vi "反应性计算.vi"(0 "首循环？":bool, 1 "λi*Ci(0)":sgl[][](array[numeric])=[[82.89727, 82.892685, 82.89905, 82.885956]], 3 "N(0)IN":sgl[](array[numeric]), 5 "βi":sgl[](array[numeric])=[0.000176, 0.001258, 0.001139, 0.002309, 0.000791, 0.000288], 7 "λi":sgl[](array[numeric])=[0.0125, 0.0306, 0.1167, 0.3133, 1.217, 3.266], 9 "中子寿命":sgl=2.3e-05, 11 "源强":sgl[](array[numeric]), 12 "采集间隔":sgl=0.05, 13 "中子注量率":dbl[](array[numeric])=[82.89727020263672, 82.89268493652344, 82.8990478515625, 82.88595581054688]) -> (2 "λi*Ci(t)":sgl[][](array[numeric]), 8 "反应性OUT":dbl[](array[numeric]))   [LabVIEW 2020]
uses:
  <vilib>/express/express arith-compare/Formula/XNode/ExpressFormulaBlockNode.xnode
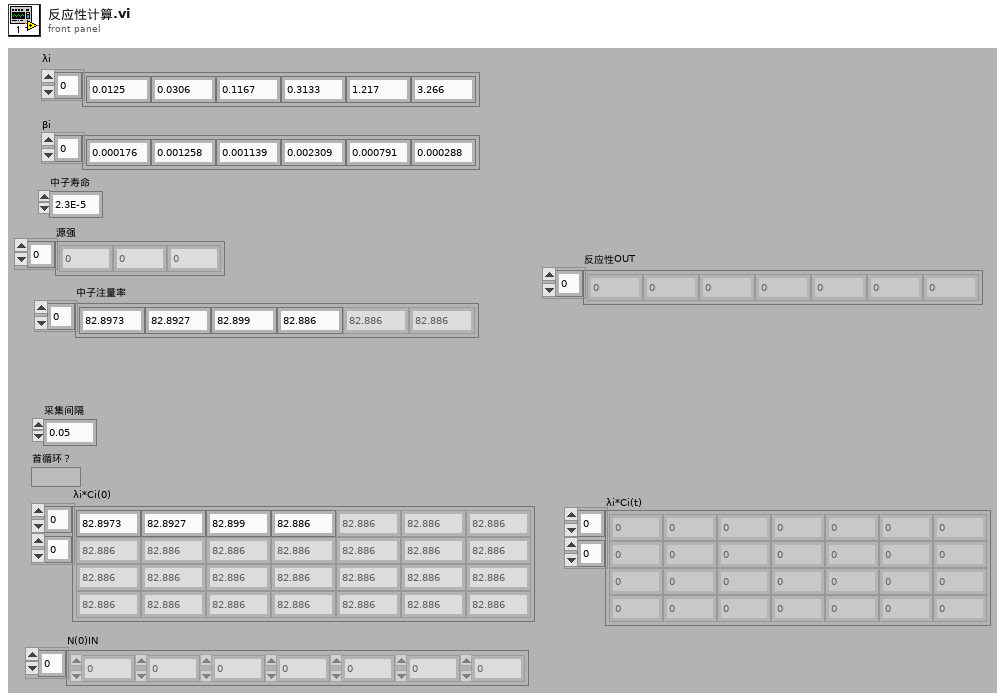
[diagram p1: front panel]
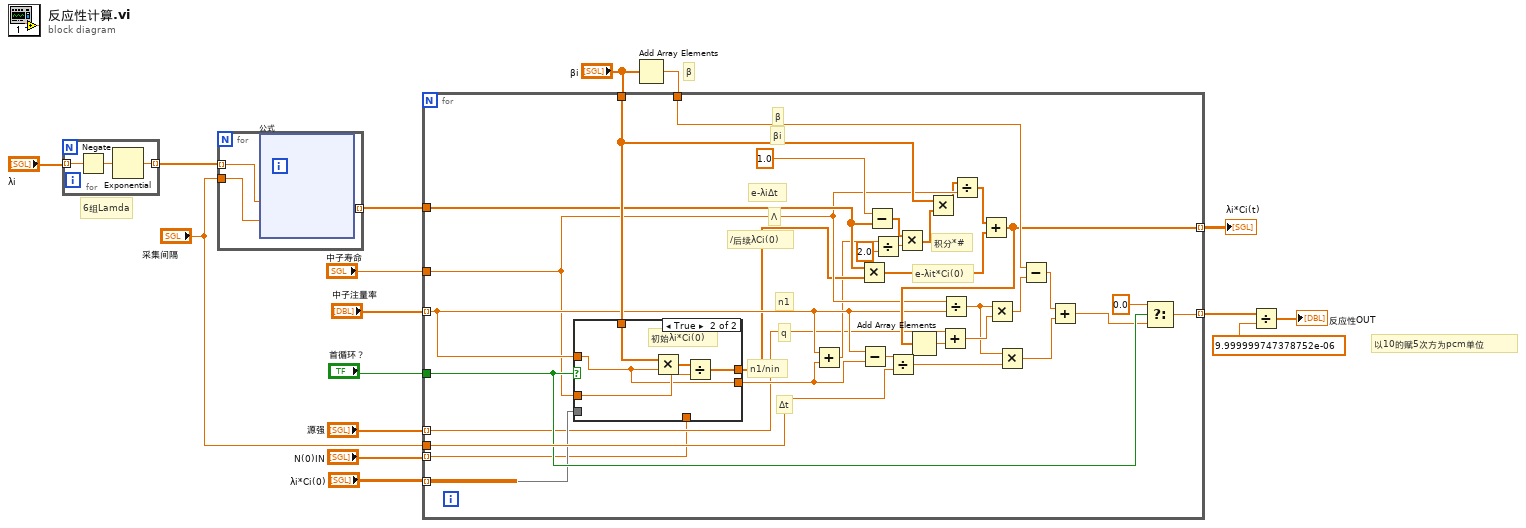
[diagram p0: block diagram]
diagram:
  # "6组Lamda"
  # "β"
  # "以10的赋5次方为pcm单位"
  n1 = for {
    tunnel: [w19] -> w6 mode=indexing
    tunnel: "λi" -> [w18] mode=indexing
    n2 = Negate(x=w18) -> (-x=w17:sgl)
    n3 = Exponential(1:w17) -> (0:w19:sgl)
  }
  n4 = for {
    tunnel: "采集间隔" -> [w21]
    tunnel: [w20] -> w5 mode=indexing
    tunnel: w6 -> [w22] mode=indexing
    n5 = xnode "公式"("X1"=w22, "X2"=w21) -> ("结果"=w20:sgl)  [unwired: 1 in, 1 out]
  }
  n6 = Add Array Elements(numeric array="βi") -> (sum=w9:sgl)
  n7 = for {
    tunnel: w9 -> [w65]
    tunnel: [w55] -> w15 mode=indexing
    tunnel: w5 -> [w54]
    tunnel: "中子注量率" -> [w60] mode=indexing
    tunnel: "βi" -> [w63]
    tunnel: "源强" -> [w34] mode=indexing
    tunnel: "中子寿命" -> [w53]
    tunnel: "λi*Ci(0)" -> [w35] mode=indexing
    tunnel: [w62] -> w13 mode=indexing
    tunnel: "首循环？" -> [w58]
    tunnel: "采集间隔" -> [w61]
    tunnel: "N(0)IN" -> [w33] mode=indexing
    # "积分*#"
    # "e-λit*Ci(0)"
    # "β"
    # "βi"
    # "n1/nin"
    # "/后续λCi(0)"
    # "q"
    # "n1"
    # "Λ"
    # "Δt"
    # "e-λiΔt"
    n8 = case shown="True" w58 {
      tunnel: w60 -> [_ w68]
      tunnel: w63 -> [_ w72]
      tunnel: [w67 w71] -> w52
      tunnel: w53 -> [_ w70]
      tunnel: w35 -> [w67 _]
      tunnel: [w66 w68] -> w59
      tunnel: w33 -> [w66 _]
      frame False {
        # "后续Ci(0)"
      }
      frame True {
        # "初始λi*Ci(0)"
        n9 = Multiply(x=w72, y=w68) -> (x*y=w69:dbl[])
        n10 = Divide(x=w69, y=w70) -> (x/y=w71:dbl[])
      }
    }
    n11 = Add(x=w60, y=w59) -> (x+y=w38:dbl)
    n12 = Multiply(x=w54, y=w52) -> (x*y=w45:dbl[])
    n13 = Subtract(x=w60, y=w59) -> (x-y=w40:dbl)
    n14 = Subtract(x=sgl 1.0, y=w54) -> (x-y=w48:sgl[])
    n15 = Divide(x=w38, y=sgl 2.0) -> (x/y=w36:dbl)
    n16 = Divide(x=w40, y=w61) -> (x/y=w41:dbl)
    n17 = Multiply(x=w48, y=w36) -> (x*y=w39:dbl[])
    n18 = Multiply(x=w63, y=w39) -> (x*y=w47:dbl[])
    n19 = Divide(x=w53, y=w60) -> (x/y=w43:dbl)
    n20 = Divide(x=w47, y=w53) -> (x/y=w46:dbl[])
    n21 = Add(x=w46, y=w45) -> (x+y=w62:dbl[])
    n22 = Add Array Elements(numeric array=w62) -> (sum=w49:dbl)
    n23 = Add(x=w34, y=w49) -> (x+y=w51:dbl)
    n24 = Multiply(x=w43, y=w51) -> (x*y=w50:dbl)
    n25 = Multiply(x=w43, y=w41) -> (x*y=w42:dbl)
    n26 = Subtract(x=w65, y=w50) -> (x-y=w44:dbl)
    n27 = Add(x=w44, y=w42) -> (x+y=w56:dbl)
    n28 = Select(t=0.0, s=w58, f=w56) -> (s? t:f=w55:dbl)
  }
  "λi*Ci(t)" <- w13
  n29 = Divide(x=w15, y=sgl 1e-05) -> (x/y=→"反应性OUT":dbl[])
